vi "Logger_GetAttributes.vi"(0 "reference in":refnum<class "Logger.lvclass">, 1 "OnlyGetDvrReference(False)":bool, 5 "Error In":errorcluster) -> (14 "reference out":refnum<class "Logger.lvclass">, 15 "Data":T1, 17 "DataRef":refnum<data-value>, 19 "Error Out":errorcluster)   [LabVIEW 2023, in "Logger.lvclass"]
uses:
  Logger.lvclass
  protected/ObjectAttributes.ctl
  <vilib>/HPS-17000/MStream_grpc_CyclerMeasurement.ctl
  Logger.lvclass/Logger.ctl
  <vilib>/HPS-17000/NI_BC_client.lvlib
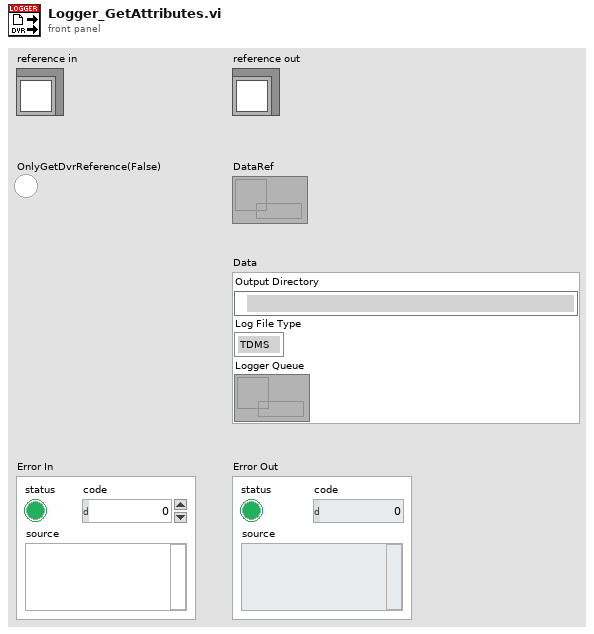
[diagram p1: front panel]
types:
  T1 = typedef "Logger.lvclass/ObjectAttributes.ctl" = cluster{"Output Directory":path, "Log File Type":enum16{"TDMS", "CSV"}, "Logger Queue":refnum<queue>}
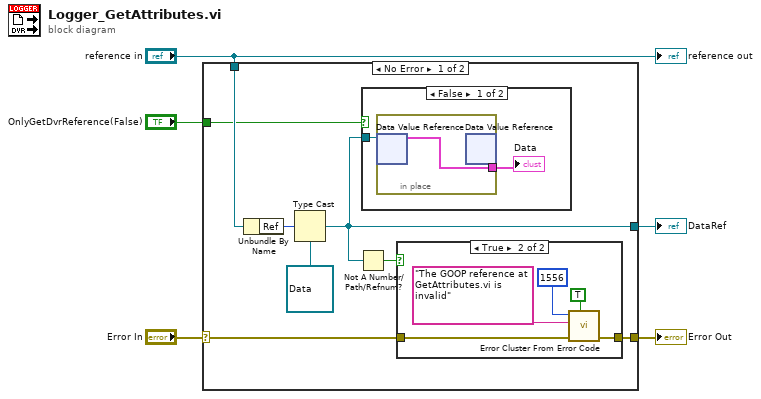
[diagram p0: block diagram]
diagram:
  n1 = case shown="No Error" "Error In" {
    selector: "Error In" -> [w13 w23]
    tunnel: [w12 w23] -> w4
    tunnel: "reference in" -> [w11 _]
    tunnel: [w10 _] -> w2
    tunnel: "OnlyGetDvrReference(False)" -> [w9 _]
    frame No Error {
      n2 = Unbundle By Name(w11) -> ("Ref"=w8:u32)
      n3 = Type Cast(type=refnum<data-value> refnum, x=w8) -> (*(type *) &x=w10:refnum<data-value>)
      n4 = Not A Number/Path/Refnum?(number/path/refnum=w10) -> (NaN/Path/Refnum?=w7:bool)
      n5 = case shown="False" w9 {
        tunnel: w10 -> [w21 _]
        frame False {
          n6 = in-place {
            in-place-border: [w22] -> w20
            n7 = in-place-dvr #1(w21) -> (w22:T1)  [unwired: 1 out]
            n8 = in-place-dvr #1() -> ()  [unwired: 1 in, 2 out]
          }
          "Data" <- w20
        }
        frame True {
        }
      }
      n9 = case shown="True" w7 {
        tunnel: w13 -> [w14 w17]
        tunnel: [w14 w16] -> w12
        frame False {
        }
        frame True {
          n10 = call <vilib>:"Error Cluster From Error Code.vi"("show call chain? (False)"=TRUE, "error in (no error)"=w17, "error message (\"\")"="The GOOP reference at GetAttributes.vi is invalid" ("source"), "error code (0)"=1556 ("code")) -> ("error out"=w16:errorcluster)  [unwired: 5 in]
        }
      }
    }
    frame Error {
    }
  }
  "Error Out" <- w4
  "DataRef" <- w2
  "reference out" <- "reference in"
